vi "Operate.vi"(8 "Error_In":errorcluster, 11 "Multiplication_In":refnum<class "Multiplication.lvclass">) -> (0 "Error_Out":errorcluster, 3 "Multiplication_Out":refnum<class "Multiplication.lvclass">)   [LabVIEW 2021, in "Multiplication.lvclass"]
doc: "Used to do Multiplication operation by over riding"
uses:
  Multiplication.lvclass
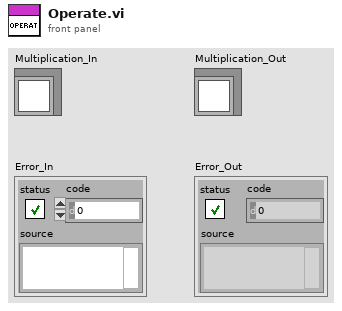
[diagram p1: front panel]
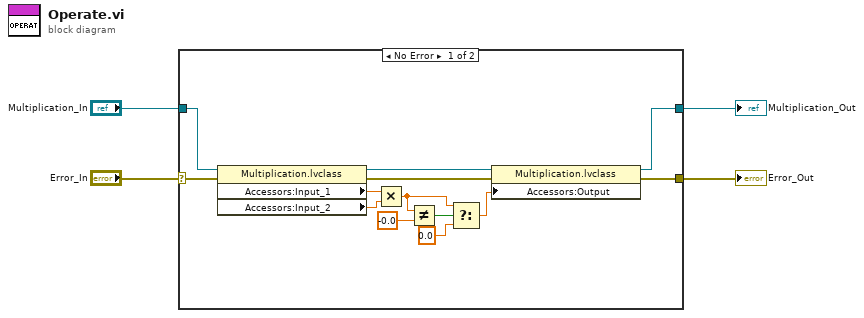
[diagram p0: block diagram]
diagram:
  n1 = case shown="No Error" "Error_In" {
    selector: "Error_In" -> [w17 w19]
    tunnel: [w15 w19] -> w1
    tunnel: [w13 w18] -> w2
    tunnel: "Multiplication_In" -> [w12 w18]
    frame No Error {
      n2 = property class="Multiplication.lvclass"(reference=w12, error in=w17) -> (reference out=w14:refnum<class "Multiplication.lvclass">, error out=w16:errorcluster, "Accessors:Input_1"=w11:dbl, "Accessors:Input_2"=w10:dbl)
      n3 = Multiply(x=w11, y=w10) -> (x*y=w9:dbl)
      n4 = Not Equal?(x=w9, y=-0.0) -> (x != y?=w8:bool)
      n5 = Select(t=w9, s=w8, f=0.0) -> (s? t:f=w7:dbl)
      n6 = property class="Multiplication.lvclass"(reference=w14, error in=w16, "Accessors:Output"=w7) -> (reference out=w13:refnum<class "Multiplication.lvclass">, error out=w15:errorcluster)
    }
    frame Error {
    }
  }
  "Error_Out" <- w1
  "Multiplication_Out" <- w2
